vi "monotone.vi"(0 "Y":dbl[](array[numeric])) -> (1 "Y2":dbl[](array[numeric]), 2 "result":bool)   [LabVIEW 2018]
panel:
  out "Boolean":bool
  out "element":dbl
  out "element 2":dbl
  out "element 3":dbl
  out "element 4":dbl
  out "element 5":dbl
  out "element 6":dbl
  out "loop_counting":dbl
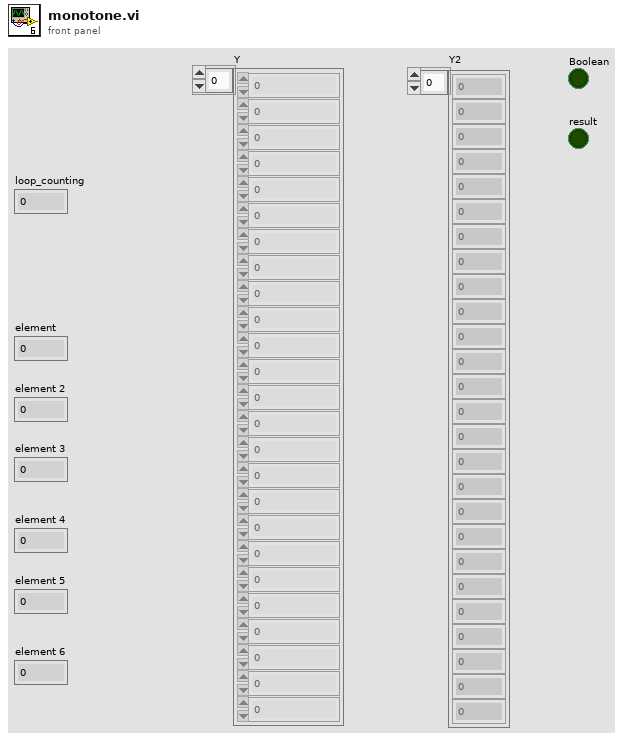
[diagram p1: front panel]
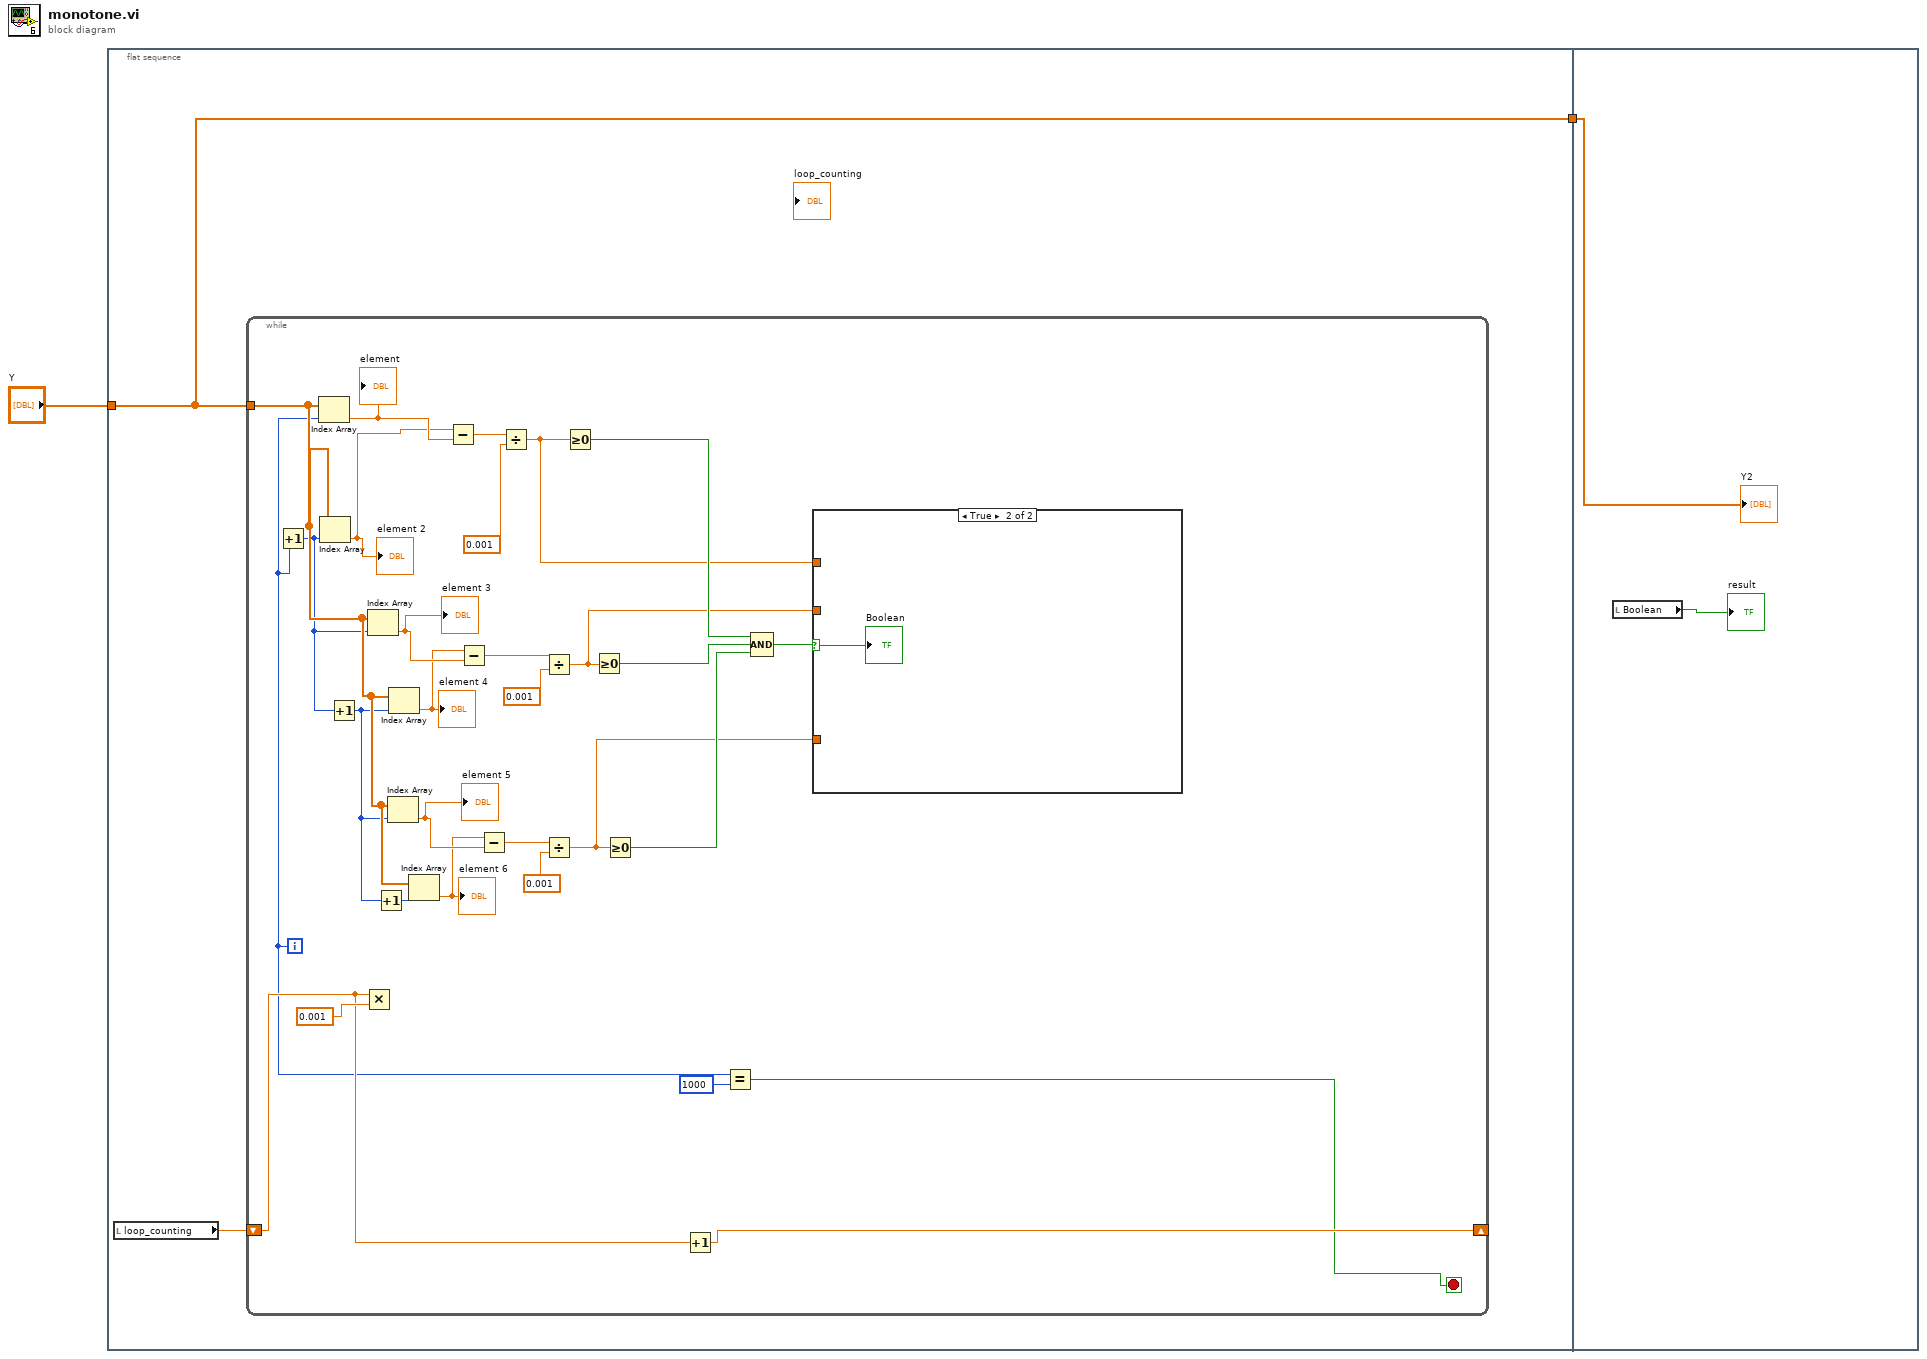
[diagram p0: block diagram]
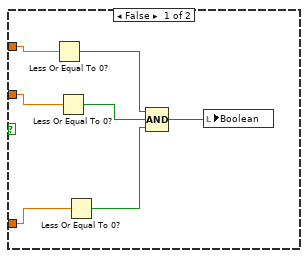
[diagram p2: hidden frame]
diagram:
  n1 = flat-sequence {
    tunnel: "Y" -> [w3]
    tunnel: [w3] -> w2
    tunnel: w2 -> [w43]
    frame #0 {
      n2 = local read "loop_counting"() -> (w4:dbl)
      n3 = while {
        tunnel: w3 -> [w22]
        shift-right: [w15] -> _
        shift-left: w4 -> [w16]
        i -> [w14]
        stop <- w12 stop-if-true
        n4 = Increment(x=w14) -> (x+1=w21:i32)
        n5 = Index Array(array=w22, index=w14) -> (element=w33:dbl)
        "element" <- w33
        n6 = Index Array(array=w22, index=w21) -> (element=w18:dbl)
        "element 2" <- w18
        n7 = Increment(x=w21) -> (x+1=w20:i32)
        n8 = Multiply(x=w16, y=0.001) -> ()  [unwired: 1 out]
        n9 = Index Array(array=w22, index=w21) -> (element=w30:dbl)
        "element 3" <- w30
        n10 = Increment(x=w20) -> (x+1=w27:i32)
        n11 = Index Array(array=w22, index=w20) -> (element=w26:dbl)
        "element 5" <- w26
        n12 = Index Array(array=w22, index=w20) -> (element=w19:dbl)
        "element 4" <- w19
        n13 = Index Array(array=w22, index=w27) -> (element=w25:dbl)
        "element 6" <- w25
        n14 = Subtract(x=w18, y=w33) -> (x-y=w32:dbl)
        n15 = Subtract(x=w19, y=w30) -> (x-y=w29:dbl)
        n16 = Subtract(x=w25, y=w26) -> (x-y=w24:dbl)
        n17 = Divide(x=w32, y=0.001) -> (x/y=w7:dbl)
        n18 = Divide(x=w29, y=0.001) -> (x/y=w6:dbl)
        n19 = Divide(x=w24, y=0.001) -> (x/y=w5:dbl)
        n20 = Greater Or Equal To 0?(x=w7) -> (x >= 0?=w11:bool)
        n21 = Greater Or Equal To 0?(x=w6) -> (x >= 0?=w10:bool)
        n22 = Greater Or Equal To 0?(x=w5) -> (x >= 0?=w9:bool)
        n23 = Increment(x=w16) -> (x+1=w15:dbl)
        n24 = Equal?(x=w14, y=1000) -> (x = y?=w12:bool)
        n25 = Compound Arithmetic op=AND(w11, w10, w9) -> (w8:bool)
        n26 = case shown="True" w8 {
          selector: w8 -> [_ w41]
          tunnel: w7 -> [w38 _]
          tunnel: w6 -> [w39 _]
          tunnel: w5 -> [w40 _]
          frame False {
            n27 = Less Or Equal To 0?(x=w38) -> (x <= 0?=w37:bool)
            n28 = Less Or Equal To 0?(x=w39) -> (x <= 0?=w36:bool)
            n29 = Less Or Equal To 0?(x=w40) -> (x <= 0?=w35:bool)
            n30 = Compound Arithmetic op=AND(w37, w36, w35) -> (w34:bool)
            n31 = local write "Boolean"(w34) -> ()
          }
          frame True {
            "Boolean" <- w41
          }
        }
      }
    }
    frame #1 {
      n32 = local read "Boolean"() -> (→"result":bool)
      "Y2" <- w43
    }
  }
